vi "Set nidaqmx_grpc_CreateCIFreqChanRequest.vi"(7 "Complete Call (T)":bool=TRUE, 8 "error in (no error)":errorcluster, 10 "package_templatemessage":T1, 11 "gRPCid":T3) -> (0 "error out":errorcluster)   [LabVIEW 2021, in "NI DAQmx_server.lvlib"]
uses:
  NI DAQmx_server.lvlib
  <vilib>/gRPC/LabVIEW gRPC Library/Shared/grpcId.ctl
  nidaqmx_grpc_CreateCIFreqChanRequest.ctl
  nidevice_grpc_Session_session/nidevice_grpc_Session_session.lvclass
  nidaqmx_grpc_CreateCIFreqChanRequest_units_enum/nidaqmx_grpc_CreateCIFreqChanRequest_units_enum.lvclass
  nidaqmx_grpc_CreateCIFreqChanRequest_edge_enum/nidaqmx_grpc_CreateCIFreqChanRequest_edge_enum.lvclass
  nidaqmx_grpc_CreateCIFreqChanRequest_meas_method_enum/nidaqmx_grpc_CreateCIFreqChanRequest_meas_method_enum.lvclass
  nidevice_grpc_Session.ctl
  nidaqmx_grpc_CreateCIFreqChanRequest_Flat.ctl
  nidevice_grpc_Session_Flat.ctl
  nidaqmx_grpc_FrequencyUnits3.ctl
  nidaqmx_grpc_Edge1.ctl
  nidaqmx_grpc_CounterFrequencyMethod.ctl
  nidevice_grpc_Session_session/nidevice_grpc_Session_session.lvclass/nidevice_grpc_Session_session.ctl
  nidaqmx_grpc_CreateCIFreqChanRequest_units_enum/nidaqmx_grpc_CreateCIFreqChanRequest_units_enum.lvclass/nidaqmx_grpc_CreateCIFreqChanRequest_units_enum.ctl
  nidaqmx_grpc_CreateCIFreqChanRequest_edge_enum/nidaqmx_grpc_CreateCIFreqChanRequest_edge_enum.lvclass/nidaqmx_grpc_CreateCIFreqChanRequest_edge_enum.ctl
  nidaqmx_grpc_CreateCIFreqChanRequest_meas_method_enum/nidaqmx_grpc_CreateCIFreqChanRequest_meas_method_enum.lvclass/nidaqmx_grpc_CreateCIFreqChanRequest_meas_method_enum.ctl
  dcc74a39-081a-4bdd-860b-8ed792803c96.vi
  RichToFlatnidevice_grpc_Session.vi
  nidaqmx_grpc_CreateCIFreqChanRequest_units_enum/GetActiveFieldIndex.vi
  nidaqmx_grpc_CreateCIFreqChanRequest_units_enum/Getunits.vi
  nidaqmx_grpc_CreateCIFreqChanRequest_units_enum/Getunits_raw.vi
  nidaqmx_grpc_CreateCIFreqChanRequest_edge_enum/GetActiveFieldIndex.vi
  nidaqmx_grpc_CreateCIFreqChanRequest_edge_enum/Getedge.vi
  nidaqmx_grpc_CreateCIFreqChanRequest_edge_enum/Getedge_raw.vi
  nidaqmx_grpc_CreateCIFreqChanRequest_meas_method_enum/GetActiveFieldIndex.vi
  nidaqmx_grpc_CreateCIFreqChanRequest_meas_method_enum/Getmeas_method.vi
  nidaqmx_grpc_CreateCIFreqChanRequest_meas_method_enum/Getmeas_method_raw.vi
  <vilib>/gRPC/LabVIEW gRPC Library/Shared/TranslateGrpcError.vi
  nidevice_grpc_Session_session/GetActiveFieldIndex.vi
  nidevice_grpc_Session_session/Getname.vi
  nidevice_grpc_Session_session/Getid.vi
  <vilib>/gRPC/LabVIEW gRPC Library/Server API/Server/Get Server DLL Path.vi
  <vilib>/Utility/error.llb/Error Cluster From Error Code.vi
  <vilib>/gRPC/LabVIEW gRPC Library/grpc-lvsupport-release.lvlib
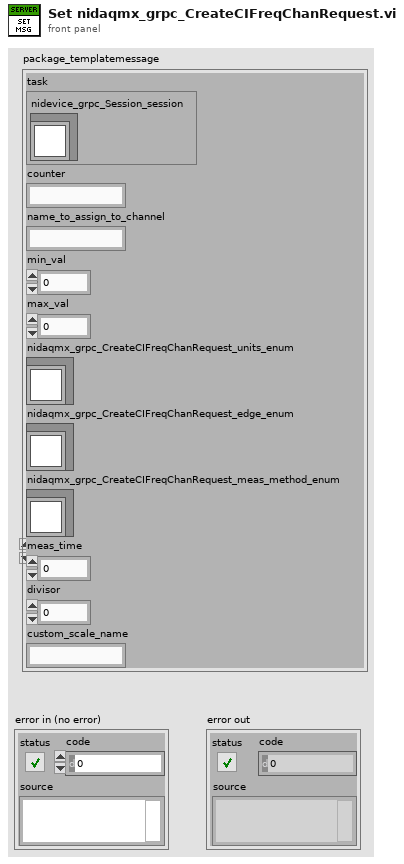
[diagram p1: front panel]
types:
  T1 = typedef "NI DAQmx_server.lvlib/nidaqmx_grpc_CreateCIFreqChanRequest.ctl" = cluster{"task":T2, "counter":string, "name_to_assign_to_channel":string, "min_val":dbl, "max_val":dbl, "nidaqmx_grpc_CreateCIFreqChanRequest_units_enum":refnum<class "nidaqmx_grpc_CreateCIFreqChanRequest_units_enum.lvclass">, "nidaqmx_grpc_CreateCIFreqChanRequest_edge_enum":refnum<class "nidaqmx_grpc_CreateCIFreqChanRequest_edge_enum.lvclass">, "nidaqmx_grpc_CreateCIFreqChanRequest_meas_method_enum":refnum<class "nidaqmx_grpc_CreateCIFreqChanRequest_meas_method_enum.lvclass">, "meas_time":dbl, "divisor":u32, "custom_scale_name":string}
  T2 = typedef "NI DAQmx_server.lvlib/nidevice_grpc_Session.ctl" = cluster{"nidevice_grpc_Session_session":refnum<class "nidevice_grpc_Session_session.lvclass">}
  T3 = typedef "grpc-lvsupport-release.lvlib/grpcId.ctl" = u64
  T4 = typedef "NI DAQmx_server.lvlib/nidaqmx_grpc_CreateCIFreqChanRequest_Flat.ctl" = cluster{"task":T5, "counter":string, "name_to_assign_to_channel":string, "min_val":dbl, "max_val":dbl, "nidaqmx_grpc_CreateCIFreqChanRequest_units_enum_selected_index":i32, "units":T6, "units_raw":i32, "nidaqmx_grpc_CreateCIFreqChanRequest_edge_enum_selected_index":i32, "edge":T7, "edge_raw":i32, "nidaqmx_grpc_CreateCIFreqChanRequest_meas_method_enum_selected_index":i32, "meas_method":T8, "meas_method_raw":i32, "meas_time":dbl, "divisor":u32, "custom_scale_name":string}
  T5 = typedef "NI DAQmx_server.lvlib/nidevice_grpc_Session_Flat.ctl" = cluster{"nidevice_grpc_Session_session_selected_index":i32, "name":string, "id":u32}
  T6 = typedef "NI DAQmx_server.lvlib/nidaqmx_grpc_FrequencyUnits3.ctl" = enum32{"FREQUENCY_UNITS3_UNSPECIFIED", "FREQUENCY_UNITS3_HZ", "FREQUENCY_UNITS3_TICKS", "FREQUENCY_UNITS3_FROM_CUSTOM_SCALE"}
  T7 = typedef "NI DAQmx_server.lvlib/nidaqmx_grpc_Edge1.ctl" = enum32{"EDGE1_UNSPECIFIED", "EDGE1_RISING", "EDGE1_FALLING"}
  T8 = typedef "NI DAQmx_server.lvlib/nidaqmx_grpc_CounterFrequencyMethod.ctl" = enum32{"COUNTER_FREQUENCY_METHOD_UNSPECIFIED", "COUNTER_FREQUENCY_METHOD_LOW_FREQ_1_CTR", "COUNTER_FREQUENCY_METHOD_HIGH_FREQ_2_CTR", "COUNTER_FREQUENCY_METHOD_LARGE_RNG_2_CTR", "COUNTER_FREQUENCY_METHOD_DYN_AVG"}
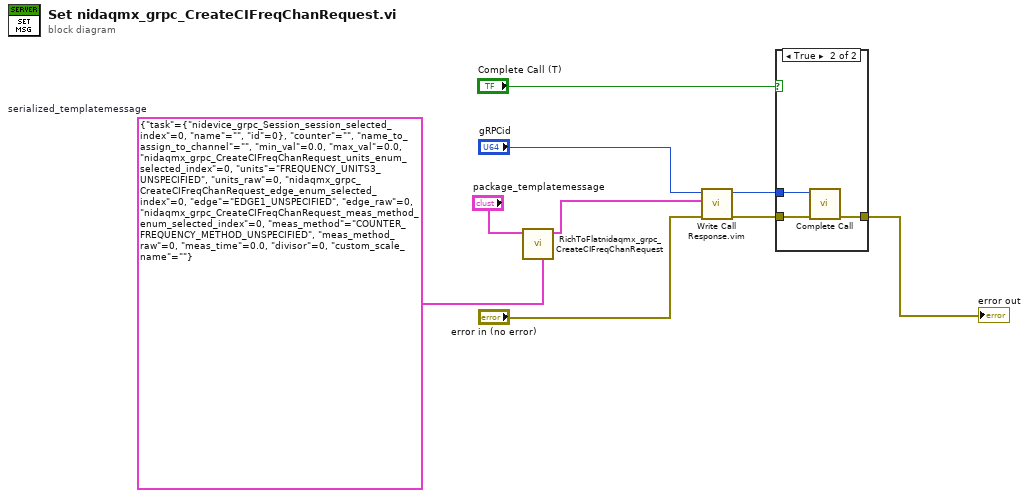
[diagram p0: block diagram]
diagram:
  w2 = T4 {"task"={"nidevice_grpc_Session_session_selected_index"=0, "name"="", "id"=0}, "counter"="", "name_to_assign_to_channel"="", "min_val"=0.0, "max_val"=0.0, "nidaqmx_grpc_CreateCIFreqChanRequest_units_enum_selected_index"=0, "units"=enum."FREQUENCY_UNITS3_UNSPECIFIED", "units_raw"=0, "nidaqmx_grpc_CreateCIFreqChanRequest_edge_enum_selected_index"=0, "edge"=enum."EDGE1_UNSPECIFIED", "edge_raw"=0, "nidaqmx_grpc_CreateCIFreqChanRequest_meas_method_enum_selected_index"=0, "meas_method"=enum."COUNTER_FREQUENCY_METHOD_UNSPECIFIED", "meas_method_raw"=0, "meas_time"=0.0, "divisor"=0, "custom_scale_name"=""}  # serialized_templatemessage
  n1 = call "RichToFlatnidaqmx_grpc_CreateCIFreqChanRequest.vi"("OutputClusterType"=w2, "InputCluster"="package_templatemessage") -> ("OutputCluster"=w1:T4)  [unwired: 9 in]
  n2 = call "Write Call Response.vim"("error in"="error in (no error)", "Response Data"=w1, "gRPCid in"="gRPCid") -> ("error out"=w6:errorcluster, "gRPCid out"=w7:T3)  [unwired: 7 in]
  n3 = case shown="True" "Complete Call (T)" {
    tunnel: [w10 w13] -> w9
    tunnel: w7 -> [_ w12]
    tunnel: w6 -> [w10 w11]
    frame False {
    }
    frame True {
      n4 = call <vilib>:"Complete Call.vi"("gRPCid"=w12, "error in"=w11) -> ("error out"=w13:errorcluster)  [unwired: 8 in]
    }
  }
  "error out" <- w9
